vi "Type Conversion.From Double (1D I8).vi"(3 "values in":dbl[](array[numeric])) -> (1 "values out":i8[](array[numeric]))   [LabVIEW 2016, in "VeriStand Data.lvlib"]
doc: "Converts the provided double float values to the specified data type, preserving the numerical value of the data."
uses:
  VeriStand Data.lvlib
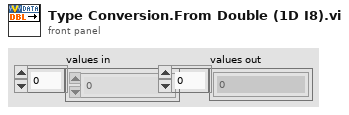
[diagram p1: front panel]
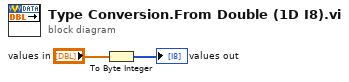
[diagram p0: block diagram]
diagram:
  n1 = To Byte Integer(number="values in") -> (8bit integer=→"values out":i8[])
